vi "Start Log.vi"(8 "error in (no error)":errorcluster, 9 "Timestamp":string, 10 "Series":string, 11 "DataLogger in":refnum<class "DataLogger.lvclass">) -> (0 "error out":errorcluster, 3 "DataLogger out":refnum<class "DataLogger.lvclass">)   [LabVIEW 2020, in "VolatusData.lvlib" / "DataLogger.lvclass"]
uses:
  DataLogger.lvclass
  DataLogger.lvclass/DataLogger.ctl
  DataHandlerTask/DataHandlerTask.lvclass
  Volatus/Task/Task.lvclass
  C:/dev/lv20CE/relink/lv-volatus/VolatusData/DataHandlerTask/DataHandlerTask.lvclass
  C:/dev/lv20CE/relink/lv-volatus/Volatus/Task/Task.lvclass
  C:/Program Files (x86)/National Instruments/LabVIEW 2020/vi.lib/ActorFramework/Actor/Actor.lvclass
  C:/dev/lv20CE/relink/lv-volatus/Volatus/TaskStateHandler/TaskStateHandler.lvclass
  C:/dev/lv20CE/relink/lv-volatus/Volatus/VectoMessageHandler/VectoMessageHandler.lvclass
  C:/dev/lv20CE/relink/lv-volatus/Volatus/API Provider/API Provider.lvclass
  C:/dev/lv20CE/relink/lv-volatus/VolatusData/DataHandler/DataHandler.lvclass
  C:/dev/lv20CE/relink/lv-volatus/VolatusData/DataLogger/DataLogger.lvclass
  C:/dev/lv20CE/relink/lv-volatus/VolatusData/LoggingHandler/LoggingHandler.lvclass
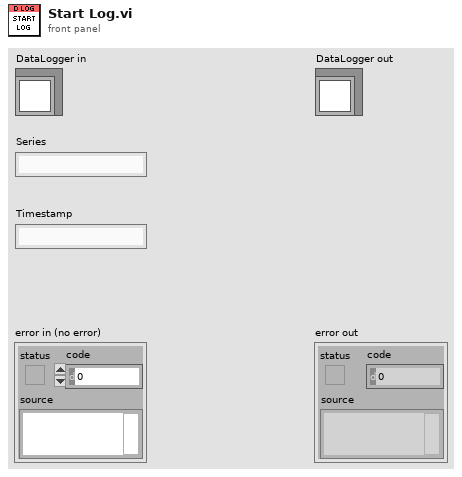
[diagram p1: front panel]
types:
  T1 = enum16{"open", "open or create", "create or replace", "create", "open (read-only)"}
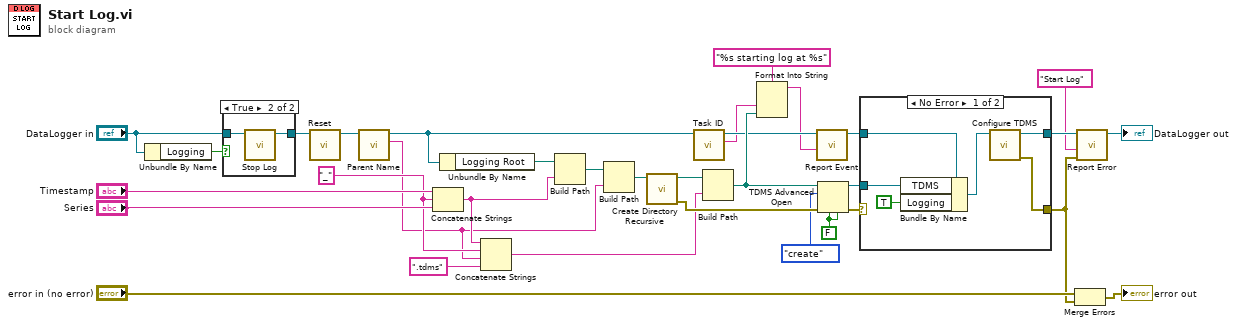
[diagram p0: block diagram]
diagram:
  w14 = FALSE
  w22 = "_" ("string")
  n1 = Unbundle By Name("DataLogger in") -> ("Logging"=w16:bool)
  n2 = case shown="True" w16 {
    tunnel: "DataLogger in" -> [w34 w36]
    tunnel: [w34 w35] -> w13
    frame False {
    }
    frame True {
      n3 = call-dynamic "Stop Log.vi"("DataLogger in"=w36) -> ("DataLogger out"=w35:refnum<class "DataLogger.lvclass">)  [unwired: 9 in, 1 out]
    }
  }
  n4 = call "Reset.vi"("DataLogger in"=w13) -> ("DataLogger out"=w19:refnum<class "DataLogger.lvclass">)  [unwired: 9 in, 1 out]
  n5 = call "Parent Name.vi"("DataHandlerTask in"=w19) -> ("Parent Name"=w11:string, "DataHandlerTask out"=w12:refnum<class "DataLogger.lvclass">)  [unwired: 8 in, 1 out]
  n6 = Concatenate Strings("Timestamp", w22, "Series") -> (w23:string)
  n7 = Unbundle By Name(w12) -> ("Logging Root"=w26:path)
  n8 = Concatenate Strings(w23, w22, w11, ".tdms" ("string")) -> (w20:string)
  n9 = Build Path(base path=w26, name or relative path=w23) -> (appended path=w25:path)
  n10 = Build Path(base path=w25, name or relative path=w11) -> (appended path=w24:path)
  n11 = call <vilib>:"Create Directory Recursive.vi"("directory"=w24) -> ("error out"=w27:errorcluster, "directory copy"=w21:path)  [unwired: 4 in, 1 out]
  n12 = call-dynamic "Task ID.vi"("DataLogger in"=w12) -> ("Task ID"=w7:string, "DataLogger out"=w8:refnum<class "DataLogger.lvclass">)  [unwired: 8 in, 1 out]
  n13 = Build Path(base path=w21, name or relative path=w20) -> (appended path=w10:path)
  n14 = Format Into String(format string="%s starting log at %s", w7, w10) -> (resulting string=w5:string)  [unwired: 2 in, 1 out]
  n15 = call "Report Event.vi"("Message"=w5, "Task in"=w8) -> ("Task out"=w6:refnum<class "DataLogger.lvclass">)  [unwired: 8 in, 1 out]
  n16 = TDMS Advanced Open(4:w14, 6:w14, 8:w27, 10:T1."create" ("operation (0:open)"), 11:w10) -> (0:w17:errorcluster, 3:w18:refnum<k34>)  [unwired: 1 out]
  n17 = case shown="No Error" w17 {
    selector: w17 -> [_ w44]
    tunnel: w6 -> [w42 w43]
    tunnel: w18 -> [w41 _]
    tunnel: [w38 w43] -> w29
    tunnel: [w37 w44] -> w2
    frame No Error {
      n18 = Bundle By Name(cluster=w42, "TDMS"=w41, "Logging"=TRUE) -> (w39:refnum<class "DataLogger.lvclass">)
      n19 = call "Configure TDMS.vi"("DataLogger in"=w39) -> ("error out"=w37:errorcluster, "DataLogger out"=w38:refnum<class "DataLogger.lvclass">)  [unwired: 9 in]
    }
    frame Error {
    }
  }
  n20 = Merge Errors("error in (no error)", w2) -> (→"error out":errorcluster)
  n21 = call "Report Error.vi"("error in (no error)"=w2, "Message"="Start Log", "Task in"=w29) -> ("Task out"=→"DataLogger out":refnum<class "DataLogger.lvclass">)  [unwired: 7 in, 1 out]
